vi "Batch_main.vi"(1 "Stop":bool=TRUE, 2 "ExpFilePath":path=path "C:/Documents and Settings/Bauerle/Mes documents/takada/HBT6/201612181913.h5") -> ()   [LabVIEW 2013]
uses:
  <vilib>/addons/h5labview2/base/hid_t.ctl
  fpga-bitfile-ref.ctl
  host-subvis/Fast_sequence/sequence slot/slot-use.ctl
  host-subvis/Fast_sequence/sequence slot/triggers.ctl
  host-subvis/Fast_sequence/sequence slot/DAC.ctl
  host-subvis/Fast_sequence/sequence slot/DAC_fastseq-offset.ctl
  host-subvis/Fast_sequence/sequence slot/timing.ctl
  host-subvis/Fast_sequence/sequence slot/jump.ctl
  <vilib>/addons/h5labview2/file/H5Fmode.ctl
  <vilib>/addons/h5labview2/base/lib_path.vi
  <vilib>/addons/h5labview2/base/H5Equery.vi
  <vilib>/FPGAPlugInAG/sbRIO-9602/niLvFpga_Close_sbRIO-9602.vi
  <vilib>/addons/h5labview2/dataset/H5Dread.llb/H5Dread.xnode
  <vilib>/addons/h5labview2/attrib/H5Aread.llb/H5Aread.xnode
  <vilib>/rvi/interface/nirviCloseFPGA/nirviCloseFPGA.xnode
  FPGA Bitfiles/fpga-clean1_FPGATarget_FPGAMAINlock-in_FC21E42C.lvbitx
  <vilib>/addons/h5labview2/attrib/H5Awrite.llb/H5Awrite.xnode
  <vilib>/addons/h5labview2/file/H5F.lvlib
  <vilib>/addons/h5labview2/dataset/H5D.lvlib
  <vilib>/addons/h5labview2/space/H5S.lvlib
panel:
  out "Temp data":sgl[][](array[numeric])
  out "Initial positions":T1(array[cluster])=[{"Name"="AWG", "kind"=7, "Value"=0.0}, {"Name"="Freq", "kind"=6, "Value"=2759965000.0}, {"Name"="Power", "kind"=6, "Value"=-40.0}, {"Name"="sus", "kind"=4, "Value"=0.29998779296875}, {"Name"="rus", "kind"=4, "Value"=0.29998779296875}, {"Name"="rls", "kind"=4, "Value"=0.29998779296875}, {"Name"="sls", "kind"=4, "Value"=0.059967041015625}, {"Name"="suq", "kind"=4, "Value"=-1.75994873046875}, {"Name"="suu", "kind"=4, "Value"=-0.749969482421875}, {"Name"="sur", "kind"=4, "Value"=-1.199951171875}, {"Name"="suc", "kind"=4, "Value"=-0.449981689453125}, {"Name"="sul", "kind"=4, "Value"=-0.89996337890625}, {"Name"="ruq", "kind"=4, "Value"=-1.699981689453125}, {"Name"="ruu", "kind"=4, "Value"=-0.749969482421875}, {"Name"="rur", "kind"=4, "Value"=-1.25}, {"Name"="ruc", "kind"=4, "Value"=-0.399932861328125}, {"Name"="rul", "kind"=4, "Value"=-0.89996337890625}, {"Name"="rlq", "kind"=4, "Value"=-1.7999267578125}, {"Name"="rlu", "kind"=4, "Value"=-0.89996337890625}, {"Name"="rlr", "kind"=4, "Value"=-1.199951171875}, {"Name"="rlc", "kind"=4, "Value"=-0.5999755859375}, {"Name"="rll", "kind"=4, "Value"=-0.749969482421875}, {"Name"="slq", "kind"=4, "Value"=-1.62506103515625}, {"Name"="slu", "kind"=4, "Value"=-0.89996337890625}, {"Name"="slr", "kind"=4, "Value"=-1.150054931640625}, {"Name"="slc", "kind"=4, "Value"=-0.449981689453125}, {"Name"="sll", "kind"=4, "Value"=-0.749969482421875}, {"Name"="tu", "kind"=4, "Value"=-0.89996337890625}, {"Name"="t", "kind"=4, "Value"=-0.89996337890625}, {"Name"="tl", "kind"=4, "Value"=-0.89996337890625}, {"Name"="4:7", "kind"=4, "Value"=-1.00006103515625}]
  in  "Buf size":i32=300
  out "Var index":u64[](array[numeric])=[0, 49, 0]
  out "start read vals":bool=TRUE
  in  "get variable\n interval (ms)":i32=300
  out "Indexes File":u64[](array[numeric])=[8, 21, 0]
  out "Finish":bool=TRUE
  in  "temp file interval (ms)":i32=600
  out "error out":errorcluster
  in  "File update interval (sec)":i32=3000000
  out "DAC_lock-in_info":T2={"Kind"=5, "Strings"=["DAC_Lock-in", "10.0.0.2", "V"], "uint64s"=[0, 1, 0, 0], "Doubles"=[1.0, 0.0, -1.0, -1.0, 50.0, 0.10000000149011612], "DAQmx take out list"=[]}
  out "Fast sequence parameters":T9={"Sequence size"=22, "IP address"="10.0.0.2", "Fast-seq-divider"=6661, "Trigger length"=300, "Sample count"=100, "Send all points?"=FALSE, "Upper limit"=1.0, "Lower limit"=-1.0, "Start ramp at"=0, "fast channels"=[{"dummy?"=FALSE, "panel"=0, "channel"=7}, {"dummy?"=FALSE, "panel"=1, "channel"=0}, {"dummy?"=FALSE, "panel"=0, "channel"=5}, {"dummy?"=FALSE, "panel"=1, "channel"=5}, {"dummy?"=FALSE, "panel"=1, "channel"=6}, {"dummy?"=FALSE, "panel"=1, "channel"=2}, {"dummy?"=FALSE, "panel"=2, "channel"=2}, {"dummy?"=FALSE, "panel"=2, "channel"=3}, {"dummy?"=FALSE, "panel"=2, "channel"=0}, {"dummy?"=FALSE, "panel"=2, "channel"=7}, {"dummy?"=FALSE, "panel"=3, "channel"=0}, {"dummy?"=FALSE, "panel"=2, "channel"=5}, {"dummy?"=FALSE, "panel"=3, "channel"=2}, {"dummy?"=FALSE, "panel"=3, "channel"=3}, {"dummy?"=FALSE, "panel"=3, "channel"=4}, {"dummy?"=FALSE, "panel"=4, "channel"=7}], "fastseq"=[{"use"=enum."triggers", "Triggers"={"triggers"={"1"=TRUE, "2"=TRUE, "3"=FALSE, "4"=FALSE}, "stop"=FALSE}, "DAC"={"FastChanNum"=0, "DAC offset"=0.0}, "timing"=0.0, "slot#"=0}, {"use"=enum."timing", "Triggers"={"triggers"={"1"=FALSE, "2"=FALSE, "3"=FALSE, "4"=FALSE}, "stop"=FALSE}, "DAC"={"FastChanNum"=0, "DAC offset"=0.0}, "timing"=1.0, "slot#"=0}, {"use"=enum."triggers", "Triggers"={"triggers"={"1"=TRUE, "2"=FALSE, "3"=FALSE, "4"=FALSE}, "stop"=FALSE}, "DAC"={"FastChanNum"=0, "DAC offset"=0.0}, "timing"=0.0, "slot#"=0}, {"use"=enum."timing", "Triggers"={"triggers"={"1"=FALSE, "2"=FALSE, "3"=FALSE, "4"=FALSE}, "stop"=FALSE}, "DAC"={"FastChanNum"=0, "DAC offset"=0.0}, "timing"=1.0, "slot#"=0}, {"use"=enum."DAC", "Triggers"={"triggers"={"1"=FALSE, "2"=FALSE, "3"=FALSE, "4"=FALSE}, "stop"=FALSE}, "DAC"={"FastChanNum"=1, "DAC offset"=0.0}, "timing"=0.0, "slot#"=0}, {"use"=enum."DAC", "Triggers"={"triggers"={"1"=FALSE, "2"=FALSE, "3"=FALSE, "4"=FALSE}, "stop"=FALSE}, "DAC"={"FastChanNum"=0, "DAC offset"=0.0}, "timing"=0.0, "slot#"=0}, {"use"=enum."DAC", "Triggers"={"triggers"={"1"=FALSE, "2"=FALSE, "3"=FALSE, "4"=FALSE}, "stop"=FALSE}, "DAC"={"FastChanNum"=4, "DAC offset"=0.0}, "timing"=0.0, "slot#"=0}, {"use"=enum."DAC", "Triggers"={"triggers"={"1"=FALSE, "2"=FALSE, "3"=FALSE, "4"=FALSE}, "stop"=FALSE}, "DAC"={"FastChanNum"=3, "DAC offset"=0.0}, "timing"=0.0, "slot#"=0}, {"use"=enum."DAC", "Triggers"={"triggers"={"1"=FALSE, "2"=FALSE, "3"=FALSE, "4"=FALSE}, "stop"=FALSE}, "DAC"={"FastChanNum"=7, "DAC offset"=0.0}, "timing"=0.0, "slot#"=0}, {"use"=enum."DAC", "Triggers"={"triggers"={"1"=FALSE, "2"=FALSE, "3"=FALSE, "4"=FALSE}, "stop"=FALSE}, "DAC"={"FastChanNum"=6, "DAC offset"=0.0}, "timing"=0.0, "slot#"=0}, {"use"=enum."DAC", "Triggers"={"triggers"={"1"=FALSE, "2"=FALSE, "3"=FALSE, "4"=FALSE}, "stop"=FALSE}, "DAC"={"FastChanNum"=10, "DAC offset"=0.0}, "timing"=0.0, "slot#"=0}, {"use"=enum."DAC", "Triggers"={"triggers"={"1"=FALSE, "2"=FALSE, "3"=FALSE, "4"=FALSE}, "stop"=FALSE}, "DAC"={"FastChanNum"=9, "DAC offset"=0.0}, "timing"=0.0, "slot#"=0}, {"use"=enum."timing", "Triggers"={"triggers"={"1"=FALSE, "2"=FALSE, "3"=FALSE, "4"=FALSE}, "stop"=FALSE}, "DAC"={"FastChanNum"=0, "DAC offset"=0.0}, "timing"=10.0, "slot#"=0}, {"use"=enum."DAC", "Triggers"={"triggers"={"1"=FALSE, "2"=FALSE, "3"=FALSE, "4"=FALSE}, "stop"=FALSE}, "DAC"={"FastChanNum"=1, "DAC offset"=0.0}, "timing"=0.0, "slot#"=0}, {"use"=enum."DAC", "Triggers"={"triggers"={"1"=FALSE, "2"=FALSE, "3"=FALSE, "4"=FALSE}, "stop"=FALSE}, "DAC"={"FastChanNum"=0, "DAC offset"=0.0}, "timing"=0.0, "slot#"=0}, {"use"=enum."DAC", "Triggers"={"triggers"={"1"=FALSE, "2"=FALSE, "3"=FALSE, "4"=FALSE}, "stop"=FALSE}, "DAC"={"FastChanNum"=4, "DAC offset"=0.0}, "timing"=0.0, "slot#"=0}, {"use"=enum."DAC", "Triggers"={"triggers"={"1"=FALSE, "2"=FALSE, "3"=FALSE, "4"=FALSE}, "stop"=FALSE}, "DAC"={"FastChanNum"=3, "DAC offset"=0.0}, "timing"=0.0, "slot#"=0}, {"use"=enum."DAC", "Triggers"={"triggers"={"1"=FALSE, "2"=FALSE, "3"=FALSE, "4"=FALSE}, "stop"=FALSE}, "DAC"={"FastChanNum"=7, "DAC offset"=0.0}, "timing"=0.0, "slot#"=0}, {"use"=enum."DAC", "Triggers"={"triggers"={"1"=FALSE, "2"=FALSE, "3"=FALSE, "4"=FALSE}, "stop"=FALSE}, "DAC"={"FastChanNum"=6, "DAC offset"=0.0}, "timing"=0.0, "slot#"=0}, {"use"=enum."DAC", "Triggers"={"triggers"={"1"=FALSE, "2"=FALSE, "3"=FALSE, "4"=FALSE}, "stop"=FALSE}, "DAC"={"FastChanNum"=10, "DAC offset"=0.0}, "timing"=0.0, "slot#"=0}, {"use"=enum."DAC", "Triggers"={"triggers"={"1"=FALSE, "2"=FALSE, "3"=FALSE, "4"=FALSE}, "stop"=FALSE}, "DAC"={"FastChanNum"=9, "DAC offset"=0.0}, "timing"=0.0, "slot#"=0}, {"use"=enum."jump", "Triggers"={"triggers"={"1"=FALSE, "2"=FALSE, "3"=FALSE, "4"=FALSE}, "stop"=FALSE}, "DAC"={"FastChanNum"=0, "DAC offset"=0.0}, "timing"=0.0, "slot#"=21}]} {"fastseq"."DAC"."DAC offset" min=-1 max=0.5; "fastseq"."DAC"."FastChanNum" max=15 step=1; "fastseq"."slot#" max=4095}
  out "Elapsed time":dbl[](array[numeric])=[2417234066.0, 52858.0]
  out "Indexes":i32[](array[numeric])=[8, 21, 0]
  out "sweep_dim":u64[](array[numeric])=[11, 61, 61]
  out "Readout parameters":T10(array[cluster])=[{"Kind"=0, "Strings"=["ADC", "", "V", "sud;rud;rld;sld", "nA;nA;nA;nA", "100.0;100.0;100.0;100.0"], "uint64s"=[5, 4, 250000, 1, 100, 10106, 1000000, 10000, 0, 1], "Doubles"=[1.0], "DAQmx take out list"=["", ""]}]
  out "Exp_params":T13={"filename"="201612181913", "ExpFilePath"=path "C:/Documents and Settings/Bauerle/Mes documents/takada/HBT6/201612181913.h5", "File Ref list"=[16777217, 33554433, 16777216, 33554432], "sweep_dim"=[11, 61, 61], "sweep_list"=["suq", "ruq", "rlq", "slq", "sur", "rur", "rlr", "slr", "suc", "ruc", "rlc", "slc"], "readout_list"=["sud", "rud", "rld", "sld"], "Sweep instrument bools"=[[0, 0], [0, 0], [0, 0], [0, 0], [0, 0], [0, 0], [0, 0], [0, 0], [0, 0], [0, 0], [0, 0], [0, 0], [0, 0], [0, 0], [0, 0], [0, 0], [0, 0], [0, 0], [0, 0], [0, 0], [0, 0], [0, 0], [0, 0], [0, 0], [0, 0], [0, 0], [0, 0], [0, 0], [0, 0], [0, 0], [0, 0], [0, 0], [0, 0], [0, 0], [0, 0], [0, 0], [0, 0], [0, 0], [0, 0], [0, 0], [0, 0]], "Read out instrument bools"=[[1, 0]], "Experimental bool list"=[TRUE, TRUE], "Initial move"=[{"Name"="None", "kind"=100, "Value"=0.0}], "FPGA Ref"=refnum, "Inst_parameters"={"ConfigFilePath"=path "\\\\10.0.0.7\\takada2/DATA/HBT6/data/Configs/conf_20161218_fc_load.h5", "Inst_list"=["ADC", "AWG", "Freq", "Power", "sus", "rus", "rls", "sls", "suq", "suu", "sur", "suc", "sul", "ruq", "ruu", "rur", "ruc", "rul", "rlq", "rlu", "rlr", "rlc", "rll", "slq", "slu", "slr", "slc", "sll", "tu", "t", "tl", "fast_sequence", "4:7", "suc_load", "sur_load", "ruc_load", "rur_load", "rlc_load", "rlr_load", "slc_load", "slr_load", "load_time"], "fast_mode"=[1, 0], "Wait_times"=[1, 1, 1, 1], "Inst_array"=[{"Kind"=0, "Strings"=["ADC", "", "V", "sud;rud;rld;sld", "nA;nA;nA;nA", "100.0;100.0;100.0;100.0"], "uint64s"=[5, 4, 250000, 1, 100, 10106, 1000000, 1, 0, 1], "Doubles"=[1.0], "DAQmx take out list"=[]}, {"Kind"=7, "Strings"=["AWG", "10.0.0.4", "", "C:\\Documents and Settings\\Bauerle\\Mes documents\\Bautze\\FPGA-clean_works_1.13.6_batchtest\\Python\\AWG", "dummy", "SAWnstrig_v4.py"], "uint64s"=[2, 0, 0, 3, 0, 0, 0, 0, 0, 0, 0, 0, 0, 0], "Doubles"=[1200000000.0, 1.0, 0.0, 1.0, 0.0, 1.0, 0.0, 1.0, 0.0, 1.0, 0.0, 1.0, 0.0], "DAQmx take out list"=[]}, {"Kind"=6, "Strings"=["Freq", "0:19", "GHz"], "uint64s"=[1, 0, 0, 0, 2, 0, 0, 0], "Doubles"=[2.0, -30.0, 200.0, 100.0, 0.0, 6.000999927520752, 9.000000318337698e-06, 30.0, -145.0], "DAQmx take out list"=[]}, {"Kind"=6, "Strings"=["Power", "0:19", "GHz"], "uint64s"=[1, 0, 1, 0, 2, 0, 0, 1], "Doubles"=[2.0, -30.0, 200.0, 100.0, 0.0, 6.000999927520752, 9.000000318337698e-06, 30.0, -145.0], "DAQmx take out list"=[]}, {"Kind"=4, "Strings"=["sus", "10.0.0.2", "mV"], "uint64s"=[0, 1], "Doubles"=[1.0, -1.0, 1.0, -1.0, 1.0], "DAQmx take out list"=[]}, {"Kind"=4, "Strings"=["rus", "10.0.0.2", "mV"], "uint64s"=[0, 2], "Doubles"=[1.0, -1.0, 1.0, -1.0, 1.0], "DAQmx take out list"=[]}, {"Kind"=4, "Strings"=["rls", "10.0.0.2", "mV"], "uint64s"=[0, 3], "Doubles"=[1.0, -1.0, 1.0, -1.0, 1.0], "DAQmx take out list"=[]}, {"Kind"=4, "Strings"=["sls", "10.0.0.2", "mV"], "uint64s"=[0, 4], "Doubles"=[1.0, -1.0, 1.0, -1.0, 1.0], "DAQmx take out list"=[]}, {"Kind"=4, "Strings"=["suq", "10.0.0.2", "V"], "uint64s"=[0, 5], "Doubles"=[0.30000001192092896, -2.0, 1.0, -1.0, 1.0], "DAQmx take out list"=[]}, {"Kind"=4, "Strings"=["suu", "10.0.0.2", "V"], "uint64s"=[0, 6], "Doubles"=[0.30000001192092896, -2.0, 1.0, -1.0, 1.0], "DAQmx take out list"=[]}, {"Kind"=4, "Strings"=["sur", "10.0.0.2", "V"], "uint64s"=[0, 7], "Doubles"=[0.30000001192092896, -2.0, 1.0, -1.0, 1.0], "DAQmx take out list"=[]}, {"Kind"=4, "Strings"=["suc", "10.0.0.2", "V"], "uint64s"=[1, 0], "Doubles"=[0.30000001192092896, -2.0, 1.0, -1.0, 1.0], "DAQmx take out list"=[]}, {"Kind"=4, "Strings"=["sul", "10.0.0.2", "V"], "uint64s"=[1, 1], "Doubles"=[0.30000001192092896, -2.0, 1.0, -1.0, 1.0], "DAQmx take out list"=[]}, {"Kind"=4, "Strings"=["ruq", "10.0.0.2", "V"], "uint64s"=[1, 2], "Doubles"=[0.30000001192092896, -2.0, 1.0, -1.0, 1.0], "DAQmx take out list"=[]}, {"Kind"=4, "Strings"=["ruu", "10.0.0.2", "V"], "uint64s"=[1, 3], "Doubles"=[0.30000001192092896, -2.0, 1.0, -1.0, 1.0], "DAQmx take out list"=[]}, {"Kind"=4, "Strings"=["rur", "10.0.0.2", "V"], "uint64s"=[1, 5], "Doubles"=[0.30000001192092896, -2.0, 1.0, -1.0, 1.0], "DAQmx take out list"=[]}, {"Kind"=4, "Strings"=["ruc", "10.0.0.2", "V"], "uint64s"=[1, 6], "Doubles"=[0.30000001192092896, -2.0, 1.0, -1.0, 1.0], "DAQmx take out list"=[]}, {"Kind"=4, "Strings"=["rul", "10.0.0.2", "V"], "uint64s"=[1, 7], "Doubles"=[0.30000001192092896, -2.0, 1.0, -1.0, 1.0], "DAQmx take out list"=[]}, {"Kind"=4, "Strings"=["rlq", "10.0.0.2", "V"], "uint64s"=[2, 0], "Doubles"=[0.30000001192092896, -2.0, 1.0, -1.0, 1.0], "DAQmx take out list"=[]}, {"Kind"=4, "Strings"=["rlu", "10.0.0.2", "V"], "uint64s"=[2, 1], "Doubles"=[0.30000001192092896, -2.0, 1.0, -1.0, 1.0], "DAQmx take out list"=[]}, {"Kind"=4, "Strings"=["rlr", "10.0.0.2", "V"], "uint64s"=[2, 2], "Doubles"=[0.30000001192092896, -2.0, 1.0, -1.0, 1.0], "DAQmx take out list"=[]}, {"Kind"=4, "Strings"=["rlc", "10.0.0.2", "V"], "uint64s"=[2, 3], "Doubles"=[0.30000001192092896, -2.0, 1.0, -1.0, 1.0], "DAQmx take out list"=[]}, {"Kind"=4, "Strings"=["rll", "10.0.0.2", "V"], "uint64s"=[2, 4], "Doubles"=[0.30000001192092896, -2.0, 1.0, -1.0, 1.0], "DAQmx take out list"=[]}, {"Kind"=4, "Strings"=["slq", "10.0.0.2", "V"], "uint64s"=[2, 5], "Doubles"=[0.30000001192092896, -2.0, 1.0, -1.0, 1.0], "DAQmx take out list"=[]}, {"Kind"=4, "Strings"=["slu", "10.0.0.2", "V"], "uint64s"=[2, 6], "Doubles"=[0.30000001192092896, -2.0, 1.0, -1.0, 1.0], "DAQmx take out list"=[]}, {"Kind"=4, "Strings"=["slr", "10.0.0.2", "V"], "uint64s"=[2, 7], "Doubles"=[0.30000001192092896, -2.0, 1.0, -1.0, 1.0], "DAQmx take out list"=[]}, {"Kind"=4, "Strings"=["slc", "10.0.0.2", "V"], "uint64s"=[3, 0], "Doubles"=[0.30000001192092896, -2.0, 1.0, -1.0, 1.0], "DAQmx take out list"=[]}, {"Kind"=4, "Strings"=["sll", "10.0.0.2", "V"], "uint64s"=[3, 1], "Doubles"=[0.30000001192092896, -2.0, 1.0, -1.0, 1.0], "DAQmx take out list"=[]}, {"Kind"=4, "Strings"=["tu", "10.0.0.2", "V"], "uint64s"=[3, 2], "Doubles"=[0.30000001192092896, -2.0, 1.0, -1.0, 1.0], "DAQmx take out list"=[]}, {"Kind"=4, "Strings"=["t", "10.0.0.2", "V"], "uint64s"=[3, 3], "Doubles"=[0.30000001192092896, -2.0, 1.0, -1.0, 1.0], "DAQmx take out list"=[]}, {"Kind"=4, "Strings"=["tl", "10.0.0.2", "V"], "uint64s"=[3, 4], "Doubles"=[0.30000001192092896, -2.0, 1.0, -1.0, 1.0], "DAQmx take out list"=[]}, {"Kind"=9, "Strings"=["fast_sequence", "10.0.0.2", "V"], "uint64s"=[6661, 300, 100, 0, 7, 8, 5, 13, 14, 10, 18, 19, 16, 23, 24, 21, 26, 27, 28, 39, 0], "Doubles"=[1.0, -1.0, -1.0, -1.0], "DAQmx take out list"=[]}, {"Kind"=4, "Strings"=["4:7", "10.0.0.2", "V"], "uint64s"=[4, 7], "Doubles"=[0.30000001192092896, -2.0, 1.0, -1.0, 1.0], "DAQmx take out list"=[]}, {"Kind"=10, "Strings"=["suc_load", "10.0.0.2", "V"], "uint64s"=[4, 0], "Doubles"=[0.5, -0.5], "DAQmx take out list"=[]}, {"Kind"=10, "Strings"=["sur_load", "10.0.0.2", "V"], "uint64s"=[5, 0], "Doubles"=[0.5, -0.5], "DAQmx take out list"=[]}, {"Kind"=10, "Strings"=["ruc_load", "10.0.0.2", "V"], "uint64s"=[6, 0], "Doubles"=[0.5, -0.5], "DAQmx take out list"=[]}, {"Kind"=10, "Strings"=["rur_load", "10.0.0.2", "V"], "uint64s"=[7, 0], "Doubles"=[0.5, -0.5], "DAQmx take out list"=[]}, {"Kind"=10, "Strings"=["rlc_load", "10.0.0.2", "V"], "uint64s"=[8, 0], "Doubles"=[0.5, -0.5], "DAQmx take out list"=[]}, {"Kind"=10, "Strings"=["rlr_load", "10.0.0.2", "V"], "uint64s"=[9, 0], "Doubles"=[0.5, -0.5], "DAQmx take out list"=[]}, {"Kind"=10, "Strings"=["slc_load", "10.0.0.2", "V"], "uint64s"=[10, 0], "Doubles"=[0.5, -0.5], "DAQmx take out list"=[]}, {"Kind"=10, "Strings"=["slr_load", "10.0.0.2", "V"], "uint64s"=[11, 0], "Doubles"=[0.5, -0.5], "DAQmx take out list"=[]}, {"Kind"=10, "Strings"=["load_time", "10.0.0.2", "ms"], "uint64s"=[12, 0], "Doubles"=[1000.0, -0.009999999776482582], "DAQmx take out list"=[]}]}} {"File Ref list" format="%.0x"}
  out "Sweep inst info":T10(array[cluster])=[{"Kind"=4, "Strings"=["suq", "10.0.0.2", "V"], "uint64s"=[0, 5], "Doubles"=[0.30000001192092896, -2.0, 1.0, -1.0, 1.0], "DAQmx take out list"=[]}, {"Kind"=4, "Strings"=["ruq", "10.0.0.2", "V"], "uint64s"=[1, 2], "Doubles"=[0.30000001192092896, -2.0, 1.0, -1.0, 1.0], "DAQmx take out list"=[]}, {"Kind"=4, "Strings"=["rlq", "10.0.0.2", "V"], "uint64s"=[2, 0], "Doubles"=[0.30000001192092896, -2.0, 1.0, -1.0, 1.0], "DAQmx take out list"=[]}, {"Kind"=4, "Strings"=["slq", "10.0.0.2", "V"], "uint64s"=[2, 5], "Doubles"=[0.30000001192092896, -2.0, 1.0, -1.0, 1.0], "DAQmx take out list"=[]}, {"Kind"=4, "Strings"=["sur", "10.0.0.2", "V"], "uint64s"=[0, 7], "Doubles"=[0.30000001192092896, -2.0, 1.0, -1.0, 1.0], "DAQmx take out list"=[]}, {"Kind"=4, "Strings"=["rur", "10.0.0.2", "V"], "uint64s"=[1, 5], "Doubles"=[0.30000001192092896, -2.0, 1.0, -1.0, 1.0], "DAQmx take out list"=[]}, {"Kind"=4, "Strings"=["rlr", "10.0.0.2", "V"], "uint64s"=[2, 2], "Doubles"=[0.30000001192092896, -2.0, 1.0, -1.0, 1.0], "DAQmx take out list"=[]}, {"Kind"=4, "Strings"=["slr", "10.0.0.2", "V"], "uint64s"=[2, 7], "Doubles"=[0.30000001192092896, -2.0, 1.0, -1.0, 1.0], "DAQmx take out list"=[]}, {"Kind"=4, "Strings"=["suc", "10.0.0.2", "V"], "uint64s"=[1, 0], "Doubles"=[0.30000001192092896, -2.0, 1.0, -1.0, 1.0], "DAQmx take out list"=[]}, {"Kind"=4, "Strings"=["ruc", "10.0.0.2", "V"], "uint64s"=[1, 6], "Doubles"=[0.30000001192092896, -2.0, 1.0, -1.0, 1.0], "DAQmx take out list"=[]}, {"Kind"=4, "Strings"=["rlc", "10.0.0.2", "V"], "uint64s"=[2, 3], "Doubles"=[0.30000001192092896, -2.0, 1.0, -1.0, 1.0], "DAQmx take out list"=[]}, {"Kind"=4, "Strings"=["slc", "10.0.0.2", "V"], "uint64s"=[3, 0], "Doubles"=[0.30000001192092896, -2.0, 1.0, -1.0, 1.0], "DAQmx take out list"=[]}]
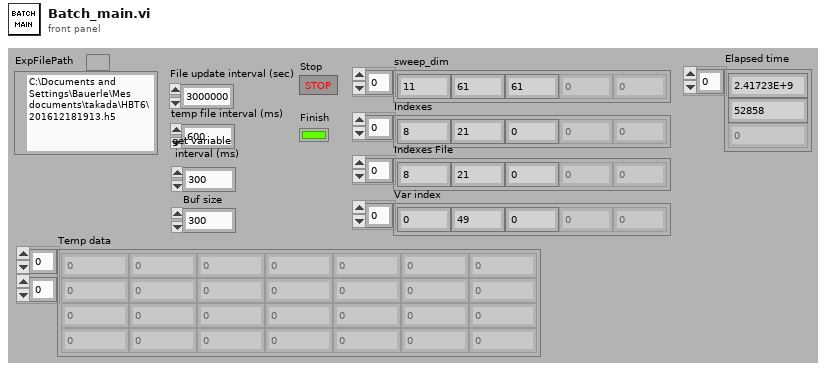
[diagram p1: front panel]
types:
  T1 = cluster{"Name":string, "kind":u64, "Value":dbl}[]
  T2 = cluster{"Kind":u16, "Strings":string[], "uint64s":u64[], "Doubles":dbl[], "DAQmx take out list":refnum<k21>[]}
  T3 = typedef "slot-use.ctl" = enum8{"DAC", "timing", "triggers", "jump"}
  T4 = typedef "triggers.ctl" = cluster{"triggers":cluster{"1":bool, "2":bool, "3":bool, "4":bool}, "stop":bool}
  T5 = typedef "DAC.ctl" = cluster{"FastChanNum":u8, "DAC offset":T6}
  T6 = typedef "DAC_fastseq-offset.ctl" = sgl
  T7 = typedef "timing.ctl" = sgl
  T8 = typedef "jump.ctl" = u16
  T9 = cluster{"Sequence size":u64, "IP address":string, "Fast-seq-divider":u64, "Trigger length":u64, "Sample count":u64, "Send all points?":bool, "Upper limit":dbl, "Lower limit":dbl, "Start ramp at":u64, "fast channels":cluster{"dummy?":bool, "panel":u8, "channel":u8}[], "fastseq":cluster{"use":T3, "Triggers":T4, "DAC":T5, "timing":T7, "slot#":T8}[]}
  T10 = cluster{"Kind":u16, "Strings":string[], "uint64s":u64[], "Doubles":dbl[], "DAQmx take out list":refnum<k21>[]}[]
  T11 = typedef "hid_t.ctl" = i32
  T12 = typedef "fpga-bitfile-ref.ctl" = refnum<k20>
  T13 = cluster{"filename":string, "ExpFilePath":path, "File Ref list":T11[], "sweep_dim":u64[], "sweep_list":string[], "readout_list":string[], "Sweep instrument bools":u64[][], "Read out instrument bools":u64[][], "Experimental bool list":bool[], "Initial move":cluster{"Name":string, "kind":u64, "Value":dbl}[], "FPGA Ref":T12, "Inst_parameters":cluster{"ConfigFilePath":path, "Inst_list":string[], "fast_mode":u8[], "Wait_times":u64[], "Inst_array":cluster{"Kind":u16, "Strings":string[], "uint64s":u64[], "Doubles":dbl[], "DAQmx take out list":refnum<k21>[]}[]}}
  T14 = cluster{"filename":string, "ExpFilePath":path, "File Ref list":T11[], "sweep_dim":u64[], "sweep_list":string[], "readout_list":string[], "Sweep instrument bools":u64[][], "Read out instrument bools":u64[][], "Experimental bool list":bool[], "Initial moves":cluster{"name":string, "parameter":u64, "value":dbl}[], "FPGA Ref":T12, "Inst_parameters":cluster{"ConfigFilePath":path, "Inst_list":string[], "fast_mode":u8[], "Wait_times":u64[], "Inst_array":cluster{"Kind":u16, "Strings":string[], "uint64s":u64[], "Doubles":dbl[], "DAQmx take out list":refnum<k21>[]}[]}}
  T15 = typedef "H5F.lvlib/H5Fmode.ctl" = enum16{"read-only", "read-write", "overwrite", "create new", "open or create"}
  T16 = enum16{"stop", "set divider", "unset ramp mode", "unset stop count", "set pulse lenght", "set ramp", "start"}
  T17 = cluster{"Kind":u16, "Strings":string[], "uint64s":u64[], "Doubles":dbl[], refnum<k21>[]}[]
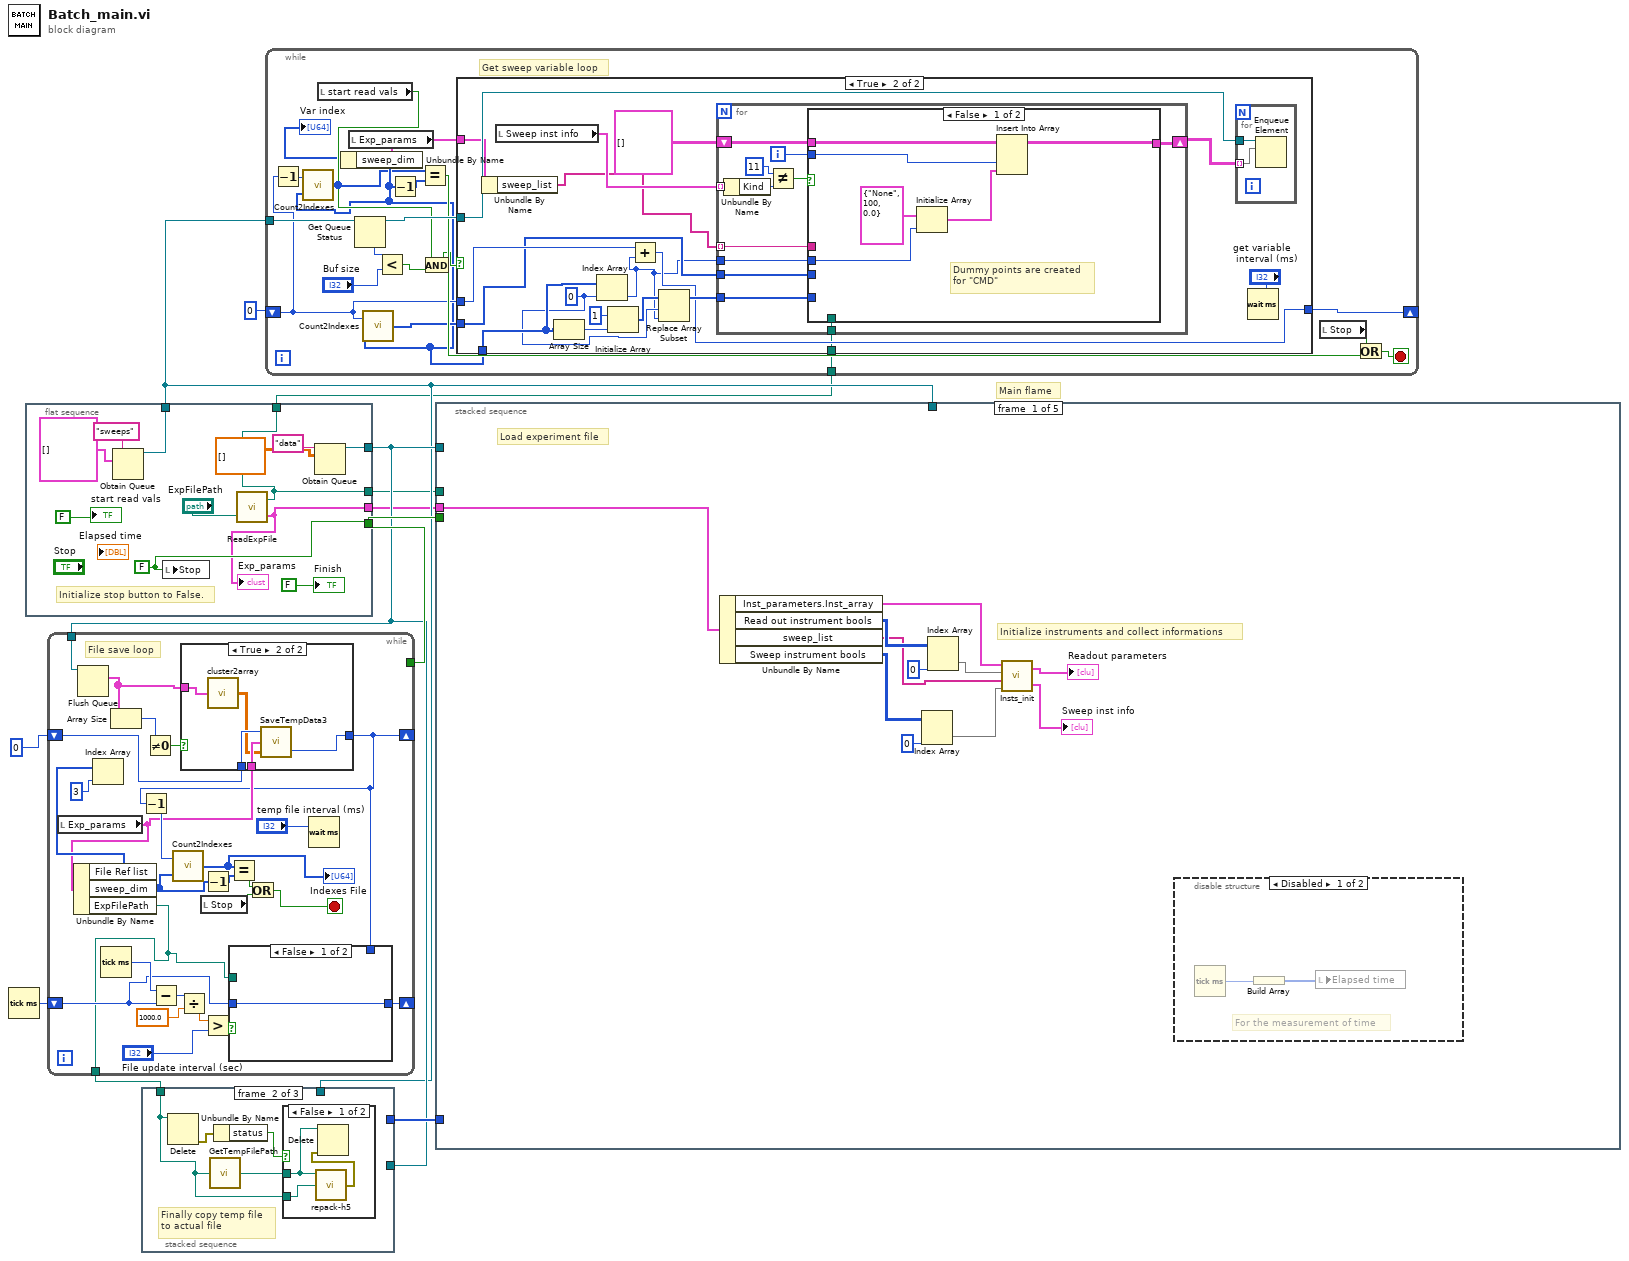
[diagram p0: block diagram]
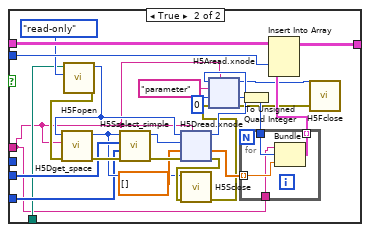
[diagram p3: hidden frame]
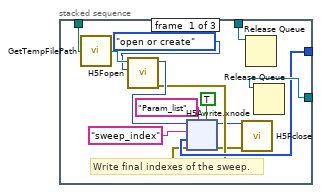
[diagram p4: hidden frame]
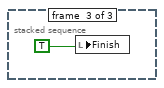
[diagram p6: hidden frame]
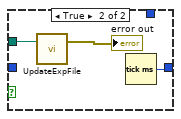
[diagram p7: hidden frame]
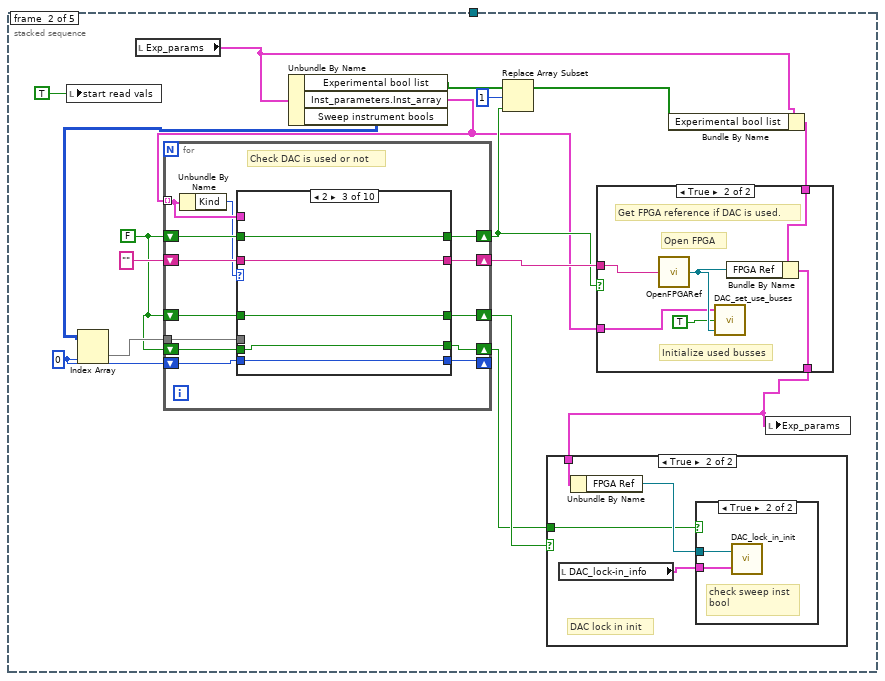
[diagram p10: hidden frame]
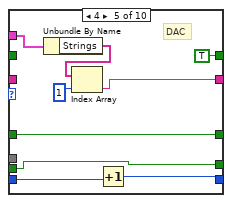
[diagram p17: hidden frame]
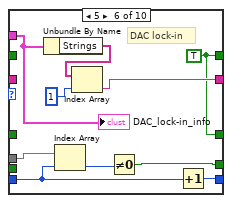
[diagram p18: hidden frame]
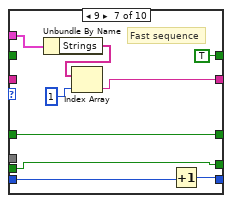
[diagram p19: hidden frame]
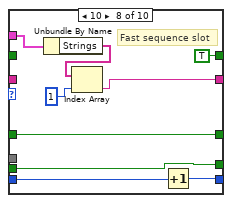
[diagram p20: hidden frame]
diagram:
  # "Main flame"
  n1 = Tick Count (ms)() -> (millisecond timer value=w10:u32)
  n2 = flat-sequence {
    tunnel: [w23] -> w7
    tunnel: [w19] -> w6
    tunnel: [w16] -> w4
    tunnel: [w13] -> w3
    tunnel: [w12] -> w2
    tunnel: [w12] -> w1
    frame #0 {
      w23 = FALSE
      # "Initialize stop button to False."
      n3 = Obtain Queue(name (unnamed)="sweeps", element data type=cluster{string, "data":u64, dbl}[] []) -> (queue out=w16:refnum<queue>)  [unwired: 3 in, 2 out]
      n4 = local write "Stop"(w23) -> ()
      n5 = call "ReadExpFile.vi"("ExpFilePath"="ExpFilePath") -> ("Exp_params"=w13:T14, "WorkFilePath"=w12:path)  [unwired: 1 in]
      "Exp_params" <- w13
      n6 = Obtain Queue(name (unnamed)="data", element data type=dbl[][] []) -> (queue out=w19:refnum<queue>)  [unwired: 3 in, 2 out]
      "Finish" <- FALSE
      "start read vals" <- FALSE
    }
  }
  n7 = while {
    shift-right: [w24] -> _
    shift-left: 0 -> [w42]
    shift-right: [w32] -> _
    shift-left: w10 -> [w33]
    tunnel: [w25] -> w8
    tunnel: w7 -> [_]
    tunnel: w6 -> [w26]
    stop <- w44 stop-if-true
    # "File save loop"
    n8 = local read "Exp_params"() -> (w29:T13)
    n9 = Unbundle By Name(w29) -> ("File Ref list"=w30:T11[], "sweep_dim"=w45:u64[], "ExpFilePath"=w25:path)
    n10 = Flush Queue(queue=w26) -> (remaining elements=w27:cluster{dbl[][]}[])  [unwired: 1 in, 2 out]
    n11 = Index Array(array=w30, index=3) -> ()  [unwired: 1 out]
    n12 = Tick Count (ms)() -> (millisecond timer value=w40:u32)
    n13 = Array Size(array=w27) -> (size(s)=w28:i32)
    n14 = Not Equal To 0?(x=w28) -> (x != 0?=w43:bool)
    n15 = Subtract(x=w40, y=w33) -> (x-y=w39:u32)
    n16 = Divide(x=w39, y=1000.0) -> (x/y=w37:dbl)
    n17 = case shown="True" w43 {
      tunnel: w42 -> [w54 w59]
      tunnel: [w54 w58] -> w24
      tunnel: w29 -> [_ w57]
      tunnel: w27 -> [_ w56]
      frame False {
      }
      frame True {
        n18 = call "cluster2array.vi"("temp data"=w56) -> ("temp data array"=w55:dbl[][][])
        n19 = call "SaveTempData3.vi"("temp data"=w55, "Exp_params"=w57, "count"=w59) -> ("count out"=w58:i32)  [unwired: 1 in]
      }
    }
    n20 = Decrement(x=w24) -> (x-1=w41:i32)
    n21 = call "Count2Indexes.vi"("sweep_dim"=w45, "Count"=w41) -> ("Indexes"=w34:u64[])
    "Indexes File" <- w34
    n22 = local read "Stop"() -> (w48:bool)
    n23 = Decrement(x=w45) -> (x-1=w46:u64[])
    n24 = Greater?(x=w37, y="File update interval (sec)") -> (0:w35:bool)
    n25 = Equal?(x=w34, y=w46) -> (x = y?=w47:bool)
    n26 = case shown="False" w35 {
      tunnel: w33 -> [w50 _]
      tunnel: [w50 w52] -> w32
      tunnel: w25 -> [_ w51]
      tunnel: w24 -> [_ _]
      frame False {
      }
      frame True {
        n27 = call "UpdateExpFile.vi"("ExpFilePath"=w51) -> ("error out"=→"error out":errorcluster)  [unwired: 2 in]
        n28 = Tick Count (ms)() -> (millisecond timer value=w52:u32)
      }
    }
    n29 = Or(x=w47, y=w48) -> (x .or. y?=w44:bool)
    n30 = Wait (ms)(milliseconds to wait="temp file interval (ms)") -> ()  [unwired: 1 out]
  }
  n31 = while {
    tunnel: w4 -> [w78]
    shift-right: [w75] -> _
    shift-left: u64 0 -> [w64]
    tunnel: w2 -> [w60]
    stop <- w72 stop-if-true
    # "Get sweep variable loop"
    n32 = Decrement(x=w64) -> (x-1=w65:u64)
    n33 = local read "start read vals"() -> (w66:bool)
    n34 = local read "Exp_params"() -> (w69:T13)
    n35 = Unbundle By Name(w69) -> ("sweep_dim"=w62:u64[])
    n36 = call "Count2Indexes.vi"("sweep_dim"=w62, "Count"=w65) -> ("Indexes"=w61:u64[])
    "Var index" <- w61
    n37 = Get Queue Status(queue=w78) -> (queue out=w74:refnum<queue>, # elements in queue=w77:i32)  [unwired: 2 in, 6 out]
    n38 = call "Count2Indexes.vi"("sweep_dim"=w62, "Count"=w64) -> ("Indexes"=w63:u64[])
    n39 = Less?(x=w77, y="Buf size") -> (x < y?=w67:bool)
    n40 = Decrement(x=w62) -> (x-1=w71:u64[])
    n41 = Equal?(x=w61, y=w71) -> (x = y?=w70:bool)
    n42 = And(x=w66, y=w67) -> (x .and. y?=w68:bool)
    n43 = case shown="True" w68 {
      tunnel: w62 -> [_ w93]
      tunnel: w64 -> [w79 w91]
      tunnel: [w79 w86] -> w75
      tunnel: w74 -> [_ w88]
      tunnel: w63 -> [_ w87]
      tunnel: w69 -> [_ w84]
      tunnel: w60 -> [_ w80]
      frame False {
      }
      frame True {
        w92 = 0
        n44 = Unbundle By Name(w84) -> ("sweep_list"=w83:string[])
        n45 = local read "Sweep inst info"() -> (w85:T10)
        n46 = Array Size(array=w93) -> (size(s)=w96:i32)
        n47 = Index Array(array=w93, index=w92) -> (element=w81:u64)
        n48 = Initialize Array(u32 1, w96) -> (w95:u32[])
        n49 = Add(x=w91, y=w81) -> (x+y=w86:u64)
        n50 = Replace Array Subset(array=w95, new element=w81, index=w92) -> (w90:u32[])
        n51 = for {
          shift-right: [w104] -> w89
          shift-left: cluster{string, "data":u16, dbl}[][] [] -> [w105]
          tunnel: w83 -> [w100] mode=indexing
          tunnel: w90 -> [w106]
          tunnel: w87 -> [w107]
          tunnel: w85 -> [w111] mode=indexing
          tunnel: w81 -> [w103]
          tunnel: w80 -> [w101]
          i -> [w102]
          n52 = Unbundle By Name(w111) -> ("Kind"=w110:u16)
          n53 = Not Equal?(x=11, y=w110) -> (x != y?=w108:bool)
          n54 = case shown="False" w108 {
            tunnel: w107 -> [_ w139]
            tunnel: w106 -> [_ w136]
            tunnel: w100 -> [_ w118]
            tunnel: w105 -> [w117 w130]
            tunnel: [w116 w129] -> w104
            tunnel: w103 -> [w114 _]
            tunnel: w102 -> [w112 w126]
            tunnel: w101 -> [_ w124]
            frame False {
              # "Dummy points are created\nfor \"CMD\""
              n55 = Initialize Array(cluster{string, "data":u64, dbl} {"None", "data"=100, 0.0}, w114) -> (w113:cluster{string, "data":u64, dbl}[])
              n56 = Insert Into Array(array=w117, index (col)=w112, new element=w113) -> (w116:cluster{string, "data":u16, dbl}[][])  [unwired: 1 in]
            }
            frame True {
              n57 = call <vilib>:"H5Fopen.vi"("mode (read-only)"=H5Fmode."read-only" ("mode"), "path"=w124) -> ("error out"=w119:errorcluster, "ref out"=w123:T11)  [unwired: 8 in]
              n58 = call <vilib>:"H5Dget_space.vi"("error in (no error)"=w119, "obj (.)"=w118, "ref in"=w123) -> ("error out"=w143:errorcluster, "space out"=w137:T11)  [unwired: 7 in]
              n59 = call <vilib>:"H5Sselect_simple.vi"("error in (no error)"=w143, "count"=w136, "start"=w139, "space in"=w137) -> ("error out"=w142:errorcluster, "space out"=w138:T11)  [unwired: 6 in]
              n60 = xnode "H5Dread.xnode"("dataset name (this)"=w118, "error in (no error)"=w142, "default"=dbl[] [], "file space"=w138, "ref in"=w123) -> ("error out"=w141:errorcluster, "data"=w135:dbl[], "ref out"=w132:T11)  [unwired: 1 in, 1 out]
              n61 = call <vilib>:"H5Sclose.vi"("error in (no error)"=w141, "space in"=w137) -> ("error out"=w122:errorcluster)  [unwired: 9 in]
              n62 = xnode "H5Aread.xnode"("object name"=w118, "error in (no error)"=w122, "default"=u16 0, "attrib name"="parameter", "ref in"=w132) -> ("error out"=w121:errorcluster, "data"=w131:u16, "ref out"=w120:T11)  [unwired: 1 in, 1 out]
              n63 = To Unsigned Quad Integer(1:w131) -> (0:w127:u64)
              n64 = for {
                tunnel: w135 -> [w162] mode=indexing
                tunnel: w127 -> [w161]
                tunnel: [w160] -> w128 mode=indexing
                tunnel: w118 -> [w159]
                n65 = Bundle(w159, w161, w162) -> (w160:cluster{string, u64, dbl})  [unwired: 1 in]
              }
              n66 = Insert Into Array(array=w130, index (col)=w126, new element=w128) -> (w129:cluster{string, "data":u16, dbl}[][])  [unwired: 1 in]
              n67 = call <vilib>:"H5Fclose.vi"("error in (no error)"=w121, "ref"=w120) -> ()  [unwired: 9 in, 1 out]
            }
          }
        }
        n68 = for {
          tunnel: w89 -> [w99] mode=indexing
          tunnel: w88 -> [w98]
          n69 = Enqueue Element(queue=w98, element=w99) -> ()  [unwired: 2 in, 3 out]
        }
        n70 = Wait (ms)(milliseconds to wait="get variable\n interval (ms)") -> ()  [unwired: 1 out]
      }
    }
    n71 = local read "Stop"() -> (w73:bool)
    n72 = Or(x=w73, y=w70) -> (x .or. y?=w72:bool)
  }
  n73 = stacked-sequence {
    tunnel: w7 -> [_ _ _ _ _]
    tunnel: [_ _ _ _ w678] -> w9
    tunnel: w6 -> [_ _ w304 _ _]
    tunnel: w4 -> [_ _ w303 _ _]
    tunnel: w3 -> [w178 _ _ _ _]
    tunnel: w1 -> [_ _ w302 w653 _]
    frame #0 {
      # "Initialize instruments and collect informations"
      # "Load experiment file"
      n74 = Unbundle By Name(w178) -> ("Inst_parameters.Inst_array"=w186:T10, "Read out instrument bools"=w185:u64[][], "sweep_list"=w183:string[], "Sweep instrument bools"=w182:u64[][])
      n75 = Index Array(array=w182, index (col)=0) -> (element=w181:u64[])  [unwired: 1 in]
      n76 = Index Array(array=w185, index (col)=0) -> (element=w184:u64[])  [unwired: 1 in]
      n77 = call "Insts_init.vi"("Initialize sweep instruments ??"=w181, "sweep_list"=w183, "Initialize readout instruments??"=w184, "Inst_array"=w186) -> ("Sweep inst parameters"=→"Sweep inst info":T17, "Readout inst parameters"=→"Readout parameters":T17)
      n78 = disable-structure shown="Disabled" {
        frame Disabled {
          # "For the measurement of time"
          n79 = Tick Count (ms)() -> (millisecond timer value=w190:u32)
          n80 = Build Array(w190) -> (w189:u32[])
          n81 = local write "Elapsed time"(w189) -> ()
        }
        frame Enabled {
        }
      }
    }
    frame #1 {
      w193 = 0
      w192 = FALSE
      n82 = local write "start read vals"(TRUE) -> ()
      n83 = local read "Exp_params"() -> (w200:T13)
      n84 = Unbundle By Name(w200) -> ("Experimental bool list"=w205:bool[], "Inst_parameters.Inst_array"=w199:T10, "Sweep instrument bools"=w195:u64[][])
      n85 = Index Array(array=w195, index (col)=w193) -> (element=w194:u64[])  [unwired: 1 in]
      n86 = for {
        tunnel: w199 -> [w230] mode=indexing
        shift-right: [w232] -> w201
        shift-left: w192 -> [w233]
        shift-right: [w229] -> w206
        shift-left: "" -> [w231]
        shift-right: [w227] -> w198
        shift-left: w192 -> [w228]
        tunnel: w194 -> [w226]
        shift-right: [w223] -> _
        shift-left: w193 -> [w224]
        shift-right: [w221] -> w191
        shift-left: w192 -> [w222]
        # "Check DAC is used or not"
        n87 = Unbundle By Name(w230) -> ("Kind"=w225:u16)
        n88 = case shown="2" w225 {
          tunnel: w233 -> [w238 w243 w248 w253 _ _ _ _ w295 w299]
          tunnel: [w238 w243 w248 w253 TRUE w268 TRUE TRUE w295 w299] -> w232
          tunnel: w231 -> [w237 w242 w247 w252 _ _ _ _ w294 w300]
          tunnel: w230 -> [_ _ _ _ w261 w272 w280 w289 _ _]
          tunnel: [w237 w242 w247 w252 w258 w269 w277 w286 w294 w300] -> w229
          tunnel: w228 -> [w236 w241 w246 w251 w257 _ w276 w285 w293 w301]
          tunnel: [w236 w241 w246 w251 w257 w268 w276 w285 w293 w301] -> w227
          tunnel: w226 -> [_ _ _ _ _ w266 _ _ _ _]
          tunnel: w224 -> [w235 w240 w245 w250 w256 w265 w274 w284 w292 w297]
          tunnel: [w235 w240 w245 w250 w255 w267 w275 w283 w292 w298] -> w223
          tunnel: [w234 w239 w244 w249 w254 w263 w273 w282 w291 w296] -> w221
          tunnel: w222 -> [w234 w239 w244 w249 w254 _ w273 w282 w291 w296]
          frame 0 {
          }
          frame 1 {
          }
          frame 2 {
          }
          frame 3 {
          }
          frame 4 {
            # "DAC"
            n89 = Unbundle By Name(w261) -> ("Strings"=w260:string[])
            n90 = Index Array(array=w260, index=1) -> (element=w258:string)
            n91 = Increment(x=w256) -> (x+1=w255:i32)
          }
          frame 5 {
            w268 = TRUE
            # "DAC lock-in"
            n92 = Unbundle By Name(w272) -> ("Strings"=w271:string[])
            n93 = Index Array(array=w266, index=w265) -> (element=w264:u64)
            n94 = Index Array(array=w271, index=1) -> (element=w269:string)
            n95 = Not Equal To 0?(x=w264) -> (x != 0?=w263:bool)
            n96 = Increment(x=w265) -> (x+1=w267:i32)
            "DAC_lock-in_info" <- w272
          }
          frame 9 {
            # "Fast sequence"
            n97 = Unbundle By Name(w280) -> ("Strings"=w279:string[])
            n98 = Index Array(array=w279, index=1) -> (element=w277:string)
            n99 = Increment(x=w274) -> (x+1=w275:i32)
          }
          frame 10 {
            # "Fast sequence slot"
            n100 = Unbundle By Name(w289) -> ("Strings"=w288:string[])
            n101 = Index Array(array=w288, index=1) -> (element=w286:string)
            n102 = Increment(x=w284) -> (x+1=w283:i32)
          }
          frame 12 {
            # "DSP lock-in readout"
          }
          frame 100, Default {
            n103 = Increment(x=w297) -> (x+1=w298:i32)
          }
        }
      }
      n104 = Replace Array Subset(array=w205, new element=w201, index=1) -> (w203:bool[])
      n105 = Bundle By Name(cluster=w200, "Experimental bool list"=w203) -> (w202:T13)
      n106 = case shown="True" w201 {
        tunnel: w206 -> [_ w220]
        tunnel: w202 -> [w214 w219]
        tunnel: [w214 w218] -> w197
        tunnel: w199 -> [_ w215]
        frame False {
        }
        frame True {
          # "Initialize used busses"
          # "Get FPGA reference if DAC is used."
          # "Open FPGA"
          n107 = call "OpenFPGARef.vi"("IP Address"=w220) -> ("FPGA VI Reference Out"=w217:T12)
          n108 = call "DAC_set_use_buses.vi"("FPGA Ref"=w217, "Use FPGA?"=TRUE, "Inst_array"=w215) -> ()  [unwired: 1 out]
          n109 = Bundle By Name(cluster=w219, "FPGA Ref"=w217) -> (w218:T13)
        }
      }
      n110 = case shown="True" w198 {
        tunnel: w197 -> [_ w211]
        tunnel: w191 -> [_ w208]
        frame False {
        }
        frame True {
          # "DAC lock in init"
          n111 = local read "DAC_lock-in_info"() -> (w209:T2)
          n112 = Unbundle By Name(w211) -> ("FPGA Ref"=w210:T12)
          n113 = case shown="True" w208 {
            tunnel: w210 -> [_ w213]
            tunnel: w209 -> [_ w212]
            frame False {
            }
            frame True {
              # "check sweep inst\nbool"
              n114 = call "DAC_lock_in_init.vi"("Inst info"=w212, "FPGA VI Reference In"=w213) -> ()  [unwired: 1 in]
            }
          }
        }
      }
      n115 = local write "Exp_params"(w197) -> ()
    }
    frame #2 {
      # "Check mode"
      n116 = local read "Exp_params"() -> (w308:T13)
      n117 = Unbundle By Name(w308) -> ("Inst_parameters.fast_mode"=w307:u8[])
      n118 = call "Sweep_mode.vi"("fast_mode"=w307) -> ("ramp?"=w305:bool, "Sweep mode"=w306:enum16{"Normal sweep", "Fast sweep"})  [unwired: 1 in]
      n119 = case shown="\"Fast sweep\"" w306 {
        tunnel: u64 0 -> [w328 w454]
        tunnel: w308 -> [w324 w444]
        tunnel: w305 -> [_ w446]
        tunnel: w304 -> [w315 w442]
        tunnel: w303 -> [w314 w441]
        tunnel: w302 -> [w311 w438]
        frame "Normal sweep", Default {
          n120 = Unbundle By Name(w324) -> ("Initial move"=w313:T1, "sweep_dim"=w323:u64[], "ExpFilePath"=w310:path, "sweep_list"=w322:string[], "Inst_parameters.Wait_times"=w321:u64[], "readout_list"=w320:string[], "FPGA Ref"=w318:T12, "Experimental bool list"=w317:bool[], "Inst_parameters.Inst_array"=w312:T10)
          n121 = local read "Readout parameters"() -> (w326:T10)
          n122 = local read "Sweep inst info"() -> (w325:T10)
          n123 = Index Array(array=w317, index=1) -> (element=w316:bool)
          n124 = stacked-sequence {
            tunnel: w328 -> [_ _ w369]
            tunnel: 0 -> [_ _ w368]
            tunnel: w326 -> [_ _ w367]
            tunnel: w325 -> [_ _ w366]
            tunnel: w323 -> [w335 _ w365]
            tunnel: w322 -> [_ _ w364]
            tunnel: w321 -> [w333 _ w363]
            tunnel: w320 -> [_ _ w362]
            tunnel: w318 -> [w332 w348 w361]
            tunnel: w316 -> [w330 w347 w360]
            tunnel: w315 -> [_ _ w359]
            tunnel: w314 -> [_ _ w358]
            tunnel: w313 -> [w334 _ _]
            tunnel: w312 -> [w331 w349 _]
            tunnel: w311 -> [w329 _ w357]
            tunnel: w310 -> [_ w346 _]
            frame #0 {
              # "Perform initial movement"
              # "Collect information of the instruments\nto be moved at the beggining."
              # "Wait after initial movement"
              n125 = Index Array(array=w333, index=0) -> (element=w337:u64)
              n126 = call "Select_inst_info.vi"("Inst_parameters.Inst_array"=w331, "Initial move"=w334) -> ("Inst_parameters.Inst_array 2"=w336:T10)
              n127 = flat-sequence {
                tunnel: w334 -> [w341]
                tunnel: w332 -> [w343]
                tunnel: w336 -> [w342]
                tunnel: w330 -> [w340]
                tunnel: w329 -> [w339]
                tunnel: w337 -> [w344]
                frame #0 {
                  # "Move"
                  n128 = call "Move.vi"("Points"=w341, "Sweep inst info"=w342, "FPGA Ref"=w343, "Use FPGA?"=w340, "WorkFilePath"=w339) -> ()  [unwired: 5 in, 1 out]
                }
                frame #1 {
                  # "Initial wait (ms)"
                  n129 = Wait (ms)(milliseconds to wait=w344) -> ()  [unwired: 1 out]
                }
              }
              "sweep_dim" <- w335
            }
            frame #1 {
              # "Register value of all the instruments before the measurement"
              n130 = call "GetTempFilePath.vi"("ExpFilePath"=w346) -> ("Temp file path"=w345:path)
              n131 = case shown="False" w347 {
                tunnel: w348 -> [_ w356]
                tunnel: [w352 w355] -> w350
                frame False {
                  w354 = 8
                  n132 = Initialize Array(0.0, w354, w354) -> (w352:dbl[][])
                }
                frame True {
                  n133 = call "DAC_current_values.vi"("FPGA Ref"=w356) -> ("DAC values"=w355:sgl[][])
                }
              }
              n134 = call "Get_values.vi"("DAC values"=w350, "Inst_array"=w349, "Temp file path"=w345) -> ("Initial positions"=→"Initial positions":T1)
            }
            frame #2 {
              n135 = while {
                shift-right: [w394] -> _
                shift-left: w369 -> [w378]
                shift-right: [w386] -> _
                shift-left: w368 -> [w387]
                tunnel: w367 -> [w384]
                tunnel: w366 -> [w377]
                tunnel: w365 -> [w383]
                tunnel: w364 -> [w372]
                tunnel: w363 -> [w382]
                tunnel: w362 -> [w381]
                tunnel: w361 -> [w380]
                tunnel: w360 -> [w379]
                tunnel: w359 -> [w376]
                tunnel: w358 -> [w375]
                tunnel: w357 -> [w370]
                stop <- w393 stop-if-true
                # "Seep indexes"
                # "Stop if stop button is pushed or\nindex reaches the sweep dimension."
                n136 = Array Size(array=w372) -> (size(s)=w373:i32)
                n137 = Not Equal To 0?(x=w373) -> (x != 0?=w371:bool)
                n138 = case shown="False" w371 {
                  tunnel: w375 -> [_ w397]
                  tunnel: [cluster{string, "data":u64, dbl}[] [{"None", "data"=100, 0.0}] w396] -> w374
                  frame False {
                  }
                  frame True {
                    n139 = Dequeue Element(queue=w397) -> (element=w396:cluster{string, "data":u64, dbl}[])  [unwired: 2 in, 3 out]
                  }
                }
                n140 = call "Count2Indexes.vi"("sweep_dim"=w383, "Count"=w378) -> ("Indexes"=w391:u64[])
                "Indexes" <- w391
                n141 = Increment(x=w378) -> (x+1=w394:u64)
                n142 = stacked-sequence {
                  seq-local: [_ _ _ w427 _ _] -> [_ _ _ _ w433 _]
                  tunnel: w377 -> [w401 _ _ _ _ _]
                  tunnel: w382 -> [_ w406 w407 w430 _ _]
                  tunnel: w384 -> [_ _ _ w428 _ _]
                  tunnel: w391 -> [w400 _ w410 _ _ w435]
                  tunnel: w383 -> [_ _ _ _ _ w436]
                  tunnel: w381 -> [_ _ _ _ _ _]
                  tunnel: [_ _ _ _ _ w436] -> w389
                  tunnel: [_ _ _ _ _ w435] -> w390
                  tunnel: w387 -> [_ _ w409 _ _ _]
                  tunnel: [_ _ w408 _ _ _] -> w386
                  tunnel: w380 -> [w403 _ _ _ _ _]
                  tunnel: w379 -> [w402 _ _ _ _ _]
                  tunnel: w378 -> [_ _ _ _ _ _]
                  tunnel: w376 -> [_ _ _ _ w434 _]
                  tunnel: w374 -> [w399 _ _ _ _ _]
                  tunnel: w370 -> [w398 _ _ _ _ _]
                  frame #0 {
                    # "Wait end of movement?"
                    # "Move to the position"
                    n143 = call "Move.vi"("Points"=w399, "Sweep inst info"=w401, "FPGA Ref"=w403, "Use FPGA?"=w402, "WorkFilePath"=w398, "Indexes"=w400) -> ()  [unwired: 4 in, 1 out]
                  }
                  frame #1 {
                    # "Wait before measurement"
                    n144 = Index Array(array=w406, index=1) -> (element=w404:u64)
                    n145 = Wait (ms)(milliseconds to wait=w404) -> ()  [unwired: 1 out]
                  }
                  frame #2 {
                    # "Extra wait time\nwhen we step."
                    # "Wait after step movement"
                    n146 = Array Size(array=w410) -> (size(s)=w412:i32)
                    n147 = Greater?(x=w412, y=1) -> (0:w413:bool)
                    n148 = case shown="True" w413 {
                      tunnel: w410 -> [_ w421]
                      tunnel: w409 -> [w414 w418]
                      tunnel: [w414 w417] -> w408
                      tunnel: w407 -> [_ w415]
                      frame False {
                      }
                      frame True {
                        n149 = Index Array(array=w421, index=1) -> (element=w416:u64)
                        n150 = Equal?(x=w416, y=w418) -> (x = y?=w419:bool)
                        n151 = case shown="False" w419 {
                          tunnel: w418 -> [_ w426]
                          tunnel: [w425 w426] -> w417
                          tunnel: w416 -> [w425 _]
                          tunnel: w415 -> [w424 _]
                          frame False {
                            n152 = Index Array(array=w424, index=3) -> (element=w422:u64)
                            n153 = Wait (ms)(milliseconds to wait=w422) -> ()  [unwired: 1 out]
                          }
                          frame True {
                          }
                        }
                      }
                    }
                  }
                  frame #3 {
                    # "Readout data"
                    n154 = Index Array(array=w430, index=2) -> (element=w429:u64)
                    n155 = call "Read.vi"("Readout parameters"=w428, "Integration time (ms)"=w429) -> ("Data"=w427:dbl[])  [unwired: 1 in]
                  }
                  frame #4 {
                    # "Save data to the file"
                    n156 = Build Array(w433) -> (w432:dbl[][])
                    n157 = local write "Temp data"(w432) -> ()
                    n158 = Enqueue Element(queue=w434, element=w432) -> ()  [unwired: 2 in, 3 out]
                  }
                  frame #5 {
                    # "Sweep counter check"
                  }
                }
                n159 = Decrement(x=w389) -> (x-1=w385:u64[])
                n160 = Equal?(x=w390, y=w385) -> (x = y?=w388:bool)
                n161 = local read "Stop"() -> (w392:bool)
                n162 = Or(x=w388, y=w392) -> (x .or. y?=w393:bool)
              }
            }
          }
        }
        frame "Fast sweep" {
          (unwired) 0
          # "File ref"
          # "Type of reding instrument\nex.) ADC, K2000, Lecroy\n(We asuume that we only\nuse 1 kind of an instrument\nat a time. If this condition is\nnot met, error comes out.)"
          # "Fast sequence size"
          # "FPGA ref"
          n163 = Unbundle By Name(w444) -> ("Initial move"=w440:T1, "FPGA Ref"=w445:T12, "Inst_parameters.ConfigFilePath"=w447:path, "sweep_dim"=w448:u64[], "sweep_list"=w451:string[], "readout_list"=w450:string[], "Inst_parameters.Wait_times"=w449:u64[], "Experimental bool list"=w443:bool[], "Inst_parameters.Inst_array"=w439:T10, "ExpFilePath"=w437:path)
          n164 = local read "Sweep inst info"() -> (w452:T10)
          n165 = local read "Readout parameters"() -> (w453:T10)
          n166 = stacked-sequence {
            seq-local: [_ w475 _ _ _ _ _] -> [_ _ w489 _ _ w558 _]
            seq-local: [w457 _ _ _ _ _ _] -> [_ w474 w487 _ _ w555 w644]
            tunnel: w454 -> [_ _ _ _ _ w564 _]
            tunnel: w453 -> [_ _ w486 _ _ _ _]
            tunnel: w452 -> [_ _ _ _ _ w561 _]
            tunnel: w451 -> [_ _ _ _ _ w562 _]
            tunnel: w450 -> [_ _ _ _ _ w557 _]
            tunnel: w449 -> [_ _ _ w528 _ w560 _]
            tunnel: w448 -> [_ _ _ w521 _ w563 _]
            tunnel: w447 -> [w463 _ _ _ _ _ _]
            tunnel: w446 -> [_ w478 w488 _ _ w559 _]
            tunnel: w445 -> [w458 _ _ w524 w543 _ _]
            tunnel: w444 -> [w462 _ _ _ _ _ _]
            tunnel: w443 -> [w460 _ _ w526 w542 w556 _]
            tunnel: w442 -> [_ _ _ _ _ w554 _]
            tunnel: w441 -> [_ _ _ _ _ w553 _]
            tunnel: w440 -> [_ _ _ w523 _ _ _]
            tunnel: w439 -> [_ _ _ w522 w541 _ _]
            tunnel: w438 -> [_ _ _ w520 _ w552 _]
            tunnel: w437 -> [_ _ _ _ w540 _ _]
            frame #0 {
              # "Get fast sequence inforamtion"
              n167 = call "Get_fast_seq_info.vi"("ConfigFilePath"=w463) -> ("Fast sequence parameters"=w456:T9)
              "Fast sequence parameters" <- w456
              n168 = Unbundle By Name(w456) -> ("IP address"=w455:string)
              n169 = Index Array(array=w460, index=1) -> (element=w459:bool)
              n170 = case shown="False" w459 {
                tunnel: w462 -> [w471 _]
                tunnel: w460 -> [w470 _]
                tunnel: w458 -> [_ w472]
                tunnel: [w465 w472] -> w457
                tunnel: w455 -> [w464 _]
                frame False {
                  # "Update use FPGA status here if it is FALSE before"
                  n171 = call "OpenFPGARef.vi"("IP Address"=w464) -> ("FPGA VI Reference Out"=w465:T12)
                  n172 = Replace Array Subset(array=w470, new element=TRUE, index=1) -> (w467:bool[])
                  n173 = Bundle By Name(cluster=w471, "Experimental bool list"=w467, "FPGA Ref"=w465) -> (w466:T13)
                  n174 = local write "Exp_params"(w466) -> ()
                }
                frame True {
                }
              }
            }
            frame #1 {
              # "Initialize the fast sequence"
              n175 = local read "Fast sequence parameters"() -> (w479:T9)
              n176 = Unbundle By Name(w479) -> ("Sequence size"=w477:u64, "Sample count"=w476:u64, "Start ramp at"=w473:u64)
              n177 = call "Fast_seq_init.vi"("FPGA Ref"=w474, "Ramp?"=w478, "Fast sequence parameters 2"=w479) -> ()
              n178 = case shown="False" w478 {
                tunnel: [w480 w481] -> w475
                tunnel: w477 -> [_ w485]
                tunnel: w476 -> [w480 _]
                tunnel: w473 -> [_ w482]
                frame False {
                }
                frame True {
                  n179 = Subtract(x=w485, y=1) -> (x-y=w483:u64)
                  n180 = Add(x=w483, y=w482) -> (x+y=w481:u64)
                }
              }
            }
            frame #2 {
              # "Configure and initialize voltmeters for fast ramp"
              n181 = for {
                tunnel: w486 -> [w495] mode=indexing
                tunnel: w489 -> [w494]
                tunnel: w488 -> [w493]
                tunnel: w487 -> [w492]
                tunnel: w486 -> [w491]
                i -> [w490]
                n182 = Unbundle By Name(w495) -> ("Kind"=w496:u16)
                n183 = case shown="12" w496 {
                  tunnel: w495 -> [w499 w508 _ w518 _]
                  tunnel: w494 -> [w504 w507 _ w516 _]
                  tunnel: w493 -> [w505 _ _ w517 _]
                  tunnel: w492 -> [_ w506 _ w519 _]
                  tunnel: w491 -> [w501 _ _ _ _]
                  tunnel: w490 -> [w500 _ _ _ _]
                  frame 0 {
                    # "Update take out\nand sample per\nchannel"
                    # "ADC"
                    n184 = local read "Fast sequence parameters"() -> (w503:T9)
                    n185 = Unbundle By Name(w503) -> ("Fast-seq-divider"=w502:u64)
                    n186 = call "ADC_config_fastsweep.vi"("Inst_parameter"=w499, "Fast sequence size"=w504, "fast sequence divider"=w502, "Ramp?"=w505) -> ("Inst_parameter out"=w497:T2)  [unwired: 1 in]
                    n187 = Replace Array Subset(array=w501, new element=w497, index=w500) -> (w498:T10)
                    n188 = local write "Readout parameters"(w498) -> ()
                  }
                  frame 1 {
                    # "K2000"
                    n189 = stacked-sequence {
                      tunnel: w508 -> [w511 w515]
                      tunnel: w507 -> [w510 _]
                      tunnel: w506 -> [w509 _]
                      frame #0 {
                        n190 = call "K2000_config_fastsweep.vi"("Readout_inst_parameters"=w511, "readings"=w510) -> ()  [unwired: 1 in, 1 out]
                        n191 = call "DAC_set_stop-sample-count.vi"("FPGA VI Reference In"=w509) -> ()  [unwired: 1 in, 10 out]
                      }
                      frame #1 {
                        n192 = Unbundle By Name(w515) -> ("Strings"=w514:string[])
                        n193 = Index Array(array=w514, index=1) -> (element=w512:string)
                        n194 = call "K2000_init_fastseq.vi"("GPIB address"=w512) -> ()
                      }
                    }
                  }
                  frame 3 {
                    # "LeCroy"
                  }
                  frame 12 {
                    # "Lock-in"
                    n195 = call "DSP_init_fast_sweep.vi"("Sample count"=w516, "ramp?"=w517, "Inst info"=w518) -> ()  [unwired: 1 in]
                    n196 = call "DAC_set_stop-sample-count.vi"("FPGA VI Reference In"=w519) -> ()  [unwired: 1 in, 10 out]
                  }
                  frame 100, Default {
                  }
                }
              }
            }
            frame #3 {
              # "Perform initial movement"
              # "Collect information of the instruments\nto be moved at the beggining."
              # "Wait after initial movement"
              n197 = local write "sweep_dim"(w521) -> ()
              n198 = Index Array(array=w526, index=1) -> (element=w525:bool)
              n199 = Index Array(array=w528, index=0) -> (element=w530:u64)
              n200 = call "Select_inst_info.vi"("Inst_parameters.Inst_array"=w522, "Initial move"=w523) -> ("Inst_parameters.Inst_array 2"=w529:T10)
              n201 = flat-sequence {
                tunnel: w523 -> [w534]
                tunnel: w524 -> [w536]
                tunnel: w529 -> [w535]
                tunnel: w525 -> [w533]
                tunnel: w520 -> [w532]
                tunnel: w530 -> [w537]
                frame #0 {
                  # "Move"
                  n202 = call "Move.vi"("Points"=w534, "Sweep inst info"=w535, "FPGA Ref"=w536, "Use FPGA?"=w533, "WorkFilePath"=w532) -> ()  [unwired: 5 in, 1 out]
                }
                frame #1 {
                  # "Initial wait (ms)"
                  n203 = Wait (ms)(milliseconds to wait=w537) -> ()  [unwired: 1 out]
                }
              }
            }
            frame #4 {
              # "Register value of all the instruments before the measurement"
              n204 = call "GetTempFilePath.vi"("ExpFilePath"=w540) -> ("Temp file path"=w539:path)
              n205 = Index Array(array=w542, index=1) -> (element=w545:bool)
              n206 = case shown="False" w545 {
                tunnel: w543 -> [_ w551]
                tunnel: [w547 w550] -> w544
                frame False {
                  w549 = 8
                  n207 = Initialize Array(0.0, w549, w549) -> (w547:dbl[][])
                }
                frame True {
                  n208 = call "DAC_current_values.vi"("FPGA Ref"=w551) -> ("DAC values"=w550:sgl[][])
                }
              }
              n209 = call "Get_values.vi"("DAC values"=w544, "Inst_array"=w541, "Temp file path"=w539) -> ("Initial positions"=w538:T1)
              n210 = local write "Initial positions"(w538) -> ()
            }
            frame #5 {
              # "Measurement loop"
              n211 = while {
                shift-right: [w589] -> _
                shift-left: w564 -> [w573]
                tunnel: w563 -> [w584]
                tunnel: w562 -> [w566]
                tunnel: w561 -> [w572]
                tunnel: w560 -> [w581]
                tunnel: w559 -> [w580]
                tunnel: w558 -> [w579]
                tunnel: w557 -> [w578]
                tunnel: w556 -> [w576]
                tunnel: w555 -> [w575]
                tunnel: w554 -> [w571]
                tunnel: w553 -> [w570]
                tunnel: w552 -> [w565]
                stop <- w588 stop-if-true
                n212 = local read "Readout parameters"() -> (w574:T10)
                n213 = Array Size(array=w566) -> (size(s)=w568:i32)
                n214 = Not Equal To 0?(x=w568) -> (x != 0?=w567:bool)
                n215 = call "Count2Indexes.vi"("sweep_dim"=w584, "Count"=w573) -> ("Indexes"=w577:u64[])
                n216 = case shown="True" w567 {
                  tunnel: w570 -> [_ w592]
                  tunnel: [cluster{string, "data":u64, dbl}[] [{"None", "data"=100, 0.0}] w591] -> w569
                  frame False {
                  }
                  frame True {
                    n217 = Dequeue Element(queue=w592) -> (element=w591:cluster{string, "data":u64, dbl}[])  [unwired: 2 in, 3 out]
                  }
                }
                n218 = stacked-sequence {
                  seq-local: [_ _ w606 _ _ _ _ _] -> [_ _ _ w618 _ w624 _ _]
                  seq-local: [_ _ _ _ w623 _ _ _] -> [_ _ _ _ _ _ w628 _]
                  tunnel: w577 -> [w595 _ _ _ _ _ _ w641]
                  tunnel: w584 -> [_ _ _ _ _ _ _ w642]
                  tunnel: [_ _ _ _ _ _ _ w642] -> w582
                  tunnel: [_ _ _ _ _ _ _ w641] -> w583
                  tunnel: w572 -> [w596 _ _ _ _ _ _ _]
                  tunnel: w581 -> [_ w603 _ _ _ _ _ _]
                  tunnel: w580 -> [_ _ w608 _ _ _ w626 _]
                  tunnel: w579 -> [_ _ w607 _ w622 _ _ _]
                  tunnel: w574 -> [_ _ _ _ _ _ w629 _]
                  tunnel: w578 -> [_ _ _ _ _ _ _ _]
                  tunnel: w576 -> [w601 _ _ _ _ _ _ _]
                  tunnel: w575 -> [w598 _ w605 _ _ _ _ _]
                  tunnel: [w597 _ _ _ _ _ _ _] -> _
                  tunnel: w573 -> [_ _ _ _ _ _ _ _]
                  tunnel: w571 -> [_ _ _ _ _ _ w627 _]
                  tunnel: w569 -> [w594 _ _ _ _ _ _ _]
                  tunnel: w565 -> [w593 _ _ _ _ _ _ _]
                  frame #0 {
                    # "Move to the point"
                    n219 = Index Array(array=w601, index=1) -> (element=w600:bool)
                    n220 = call "Move.vi"("Points"=w594, "Sweep inst info"=w596, "FPGA Ref"=w598, "Use FPGA?"=w600, "WorkFilePath"=w593, "Indexes"=w595) -> ("FPGA VI Reference Out"=w597:T12)  [unwired: 4 in]
                  }
                  frame #1 {
                    # "Wait after step movement\n(For the fast sequence there is no wait\nbetween sweep measurement)"
                    n221 = Index Array(array=w603, index=3) -> (element=w602:u64)
                    n222 = Wait (ms)(milliseconds to wait=w602) -> ()  [unwired: 1 out]
                  }
                  frame #2 {
                    # "Start fast sequence at the new sweep"
                    n223 = case shown="False" w608 {
                      tunnel: w607 -> [w611 w613]
                      tunnel: [w610 w615] -> w606
                      tunnel: w605 -> [w609 w616]
                      frame False {
                        n224 = call "DAC_set_stop-sample-count.vi"("sample count"=w611, "FPGA VI Reference In"=w609) -> ("FPGA VI Reference Out"=w610:T12)  [unwired: 9 out]
                      }
                      frame True {
                        n225 = Add(x=w613, y=2) -> (x+y=w614:u64)
                        n226 = call "fastseq_set_orders.vi"("FPGA VI Reference In"=w616, "sample count"=w614, "Enum"=T16."set ramp") -> ("FPGA VI Reference Out"=w615:T12)  [unwired: 2 in]
                      }
                    }
                  }
                  frame #3 {
                    # "Start fast sequence"
                    n227 = call "fastseq_set_orders.vi"("FPGA VI Reference In"=w618, "Enum"=T16."start") -> ()  [unwired: 3 in, 1 out]
                  }
                  frame #4 {
                    # "Further decrease for ramp mode\n(-1 before is to remove trigger's\ncontribution and this -1 is to remove\njump contribution)."
                    # "Read data"
                    n228 = local read "Readout parameters"() -> (w621:T10)
                    n229 = call "Read_fastseq.vi"("Sequence size"=w622, "Readout parameters"=w621) -> ("measures"=w623:sgl[][], "Readout parameters out"=w620:T10)  [unwired: 2 in]
                    "Temp data" <- w623
                    n230 = local write "Readout parameters"(w620) -> ()
                  }
                  frame #5 {
                    # "Stop fast sequence"
                    n231 = call "fastseq_set_orders.vi"("FPGA VI Reference In"=w624, "Enum"=T16."stop") -> ()  [unwired: 3 in, 1 out]
                  }
                  frame #6 {
                    # "Save array data"
                    # "Clear buffer before going to next"
                    n232 = for {
                      tunnel: w629 -> [w633] mode=indexing
                      tunnel: w629 -> [w632]
                      tunnel: w626 -> [w630]
                      i -> [w631]
                      n233 = Unbundle By Name(w633) -> ("Kind"=w634:u16)
                      n234 = case shown="12" w634 {
                        tunnel: w633 -> [w638 w639 _]
                        tunnel: w632 -> [w637 _ _]
                        tunnel: w631 -> [w636 _ _]
                        tunnel: w630 -> [_ w640 _]
                        frame 0 {
                          n235 = call "ADC_clean_buffer_batch.vi"("Index"=w636, "Readout parameters in"=w637, "Inst_param_in"=w638) -> ("Readout parameters out"=w635:T10)
                          n236 = local write "Readout parameters"(w635) -> ()
                        }
                        frame 12 {
                          n237 = call "DSPClearBuffer.vi"("Inst info"=w639, "ramp?"=w640) -> ()  [unwired: 1 in]
                        }
                        frame 100, Default {
                        }
                      }
                    }
                    n238 = Enqueue Element(queue=w627, element=w628) -> ()  [unwired: 2 in, 3 out]
                  }
                  frame #7 {
                  }
                }
                n239 = Increment(x=w573) -> (x+1=w589:u64)
                n240 = local write "Indexes"(w577) -> ()
                n241 = Decrement(x=w582) -> (x-1=w585:u64[])
                n242 = local read "Stop"() -> (w587:bool)
                n243 = Equal?(x=w583, y=w585) -> (x = y?=w586:bool)
                n244 = Or(x=w586, y=w587) -> (x .or. y?=w588:bool)
              }
            }
            frame #6 {
              # "Post sweep treatment for the readout instruments"
              # "Final wait and close ADC etc."
              n245 = local read "Readout parameters"() -> (w643:T10)
              n246 = call "DAC_wait_end-of-move.vi"("FPGA VI Reference In"=w644) -> ()  [unwired: 1 in, 10 out]
              n247 = for {
                tunnel: w643 -> [w645] mode=indexing
                n248 = Unbundle By Name(w645) -> ("Kind"=w646:u16)
                n249 = case shown="100, Default" w646 {
                  tunnel: w645 -> [w652 _]
                  frame 0 {
                    w651 = 0
                    n250 = Unbundle By Name(w652) -> ("DAQmx take out list"=w649:refnum<k21>[])
                    n251 = Increment(x=w651) -> (x+1=w650:i32)
                    n252 = Index Array(array=w649, index=w651) -> (element=w648:refnum<k21>)
                    n253 = Index Array(array=w649, index=w650) -> (element=w647:refnum<k21>)
                    n254 = call <vilib>:"DAQmx Clear Task.vi"("task in"=w648) -> ()  [unwired: 14 in, 1 out]
                    n255 = call <vilib>:"DAQmx Clear Task.vi"("task in"=w647) -> ()  [unwired: 14 in, 1 out]
                  }
                  frame 100, Default {
                  }
                }
              }
            }
          }
        }
      }
    }
    frame #3 {
      # "Post measurement treatment (temporal because it is not so nice.)"
      # "Go back to the initial position if it is required."
      n256 = local read "Exp_params"() -> (w661:T13)
      n257 = Unbundle By Name(w661) -> ("Experimental bool list"=w662:bool[], "FPGA Ref"=w663:T12)
      n258 = Index Array(array=w662, index=0) -> (element=w664:bool)
      n259 = Unbundle By Name(w661) -> ("Inst_parameters.Inst_array"=w656:T10, "Read out instrument bools"=w657:u64[][], "Sweep instrument bools"=w660:u64[][])
      n260 = case shown="True" w664 {
        tunnel: w661 -> [_ w673]
        tunnel: w663 -> [_ w672]
        tunnel: w662 -> [_ w670]
        tunnel: w653 -> [_ w666]
        frame False {
        }
        frame True {
          # "Move"
          # "Get initial values of sweep"
          # "Go to initial position"
          n261 = Unbundle By Name(w673) -> ("sweep_dim"=w676:u64[], "sweep_list"=w675:string[])
          n262 = call "Count2Indexes.vi"("sweep_dim"=w676, "Count"=0) -> ("Indexes"=w667:u64[])
          n263 = local read "Sweep inst info"() -> (w668:T10)
          n264 = call "GetValueFromIndexes.vi"("sweep_list"=w675, "WorkFilePath"=w666, "Sweep inst info"=w668, "Indexes"=w667) -> ("Points"=w674:cluster{"name":string, "data":u64, "data":dbl}[])
          n265 = Index Array(array=w670, index=1) -> (element=w669:bool)
          n266 = call "Move.vi"("Points"=w674, "Sweep inst info"=w668, "FPGA Ref"=w672, "Use FPGA?"=w669, "WorkFilePath"=w666, "Indexes"=w667) -> ()  [unwired: 4 in, 1 out]
        }
      }
      n267 = Index Array(array=w660, index (col)=1) -> (element=w654:u64[])  [unwired: 1 in]
      n268 = Index Array(array=w657, index (col)=1) -> (element=w655:u64[])  [unwired: 1 in]
      n269 = call "Insts_post.vi"("Initialize sweep instruments ??"=w654, "Initialize readout instruments??"=w655, "Inst_array"=w656) -> ()  [unwired: 3 in]
    }
    frame #4 {
      n270 = local read "Indexes"() -> (w678:i32[])
      n271 = disable-structure shown="Disabled" {
        frame Disabled {
          # "Measure total time of the measurement."
          n272 = local read "Elapsed time"() -> (w685:dbl[])
          n273 = call "Timer.vi"("Elapsed time"=w685) -> ("Ellapsed time out"=w684:dbl[])
          n274 = local write "Elapsed time"(w684) -> ()
        }
        frame Enabled {
        }
      }
      n275 = local read "Exp_params"() -> (w683:T13)
      n276 = Unbundle By Name(w683) -> ("Experimental bool list"=w681:bool[], "FPGA Ref"=w682:T12)
      n277 = Index Array(array=w681, index=1) -> (element=w680:bool)
      n278 = case shown="True" w680 {
        tunnel: w682 -> [_ w686]
        frame False {
        }
        frame True {
          # "Close FPGA"
          n279 = xnode "Close FPGA VI Reference"("FPGA VI Reference In"=w686) -> ()  [unwired: 1 in, 1 out]
        }
      }
    }
  }
  n280 = stacked-sequence {
    tunnel: w9 -> [w690 _ _]
    tunnel: w8 -> [w697 w718 _]
    tunnel: w6 -> [w699 _ _]
    tunnel: w4 -> [w698 _ _]
    frame #0 {
      # "Write final indexes of the sweep."
      n281 = call "GetTempFilePath.vi"("ExpFilePath"=w697) -> ("Temp file path"=w696:path)
      n282 = call <vilib>:"H5Fopen.vi"("mode (read-only)"=H5Fmode."open or create" ("mode"), "path"=w696) -> ("error out"=w689:errorcluster, "ref out"=w691:T11)  [unwired: 8 in]
      n283 = xnode "H5Awrite.xnode"("replace? (T)"=TRUE, "object name"="Param_list", "error in (no error)"=w689, "data"=w690, "attrib name"="sweep_index", "ref in"=w691) -> ("error out"=w688:errorcluster, "ref out"=w687:T11)  [unwired: 1 in, 1 out]
      n284 = call <vilib>:"H5Fclose.vi"("error in (no error)"=w688, "ref"=w687) -> ()  [unwired: 9 in, 1 out]
      n285 = Release Queue(queue=w698) -> ()  [unwired: 2 in, 3 out]
      n286 = Release Queue(queue=w699) -> ()  [unwired: 2 in, 3 out]
    }
    frame #1 {
      # "Finally copy temp file\nto actual file"
      n287 = Delete(path (use dialog)=w718) -> (error out=w720:errorcluster)  [unwired: 4 in, 2 out]
      n288 = call "GetTempFilePath.vi"("ExpFilePath"=w718) -> ("Temp file path"=w719:path)
      n289 = Unbundle By Name(w720) -> ("status"=w721:bool)
      n290 = case shown="False" w721 {
        tunnel: w719 -> [w722 _]
        tunnel: w718 -> [w724 _]
        frame False {
          n291 = call "repack-h5.vi"("dest"=w724, "source"=w722) -> ("error out"=w723:errorcluster)  [unwired: 1 in]
          n292 = Delete(path (use dialog)=w722, error in=w723) -> ()  [unwired: 3 in, 3 out]
        }
        frame True {
        }
      }
    }
    frame #2 {
      n293 = local write "Finish"(TRUE) -> ()
    }
  }
